vi "Begin.vi"(8 "error in":errorcluster) -> (0 "error out":errorcluster)   [LabVIEW 2018]
doc: "Called before other user functions, this VI can be used to open I/O refnums, load in file data, and do general program initialization. Notice that the <B>error out</B> terminal is simply used for data flow. Wiring it to other structures or subVIs ensures that this VI runs first."
uses:
  <vilib>/Rock Robotics/WPI/DriverStation/WPI_DriverStationRobotMode2.ctl
  <vilib>/Rock Robotics/WPI/Joystick/WPI_JoystickDeviceEnum.ctl
  <vilib>/Rock Robotics/WPI/SafetyOutput/WPI_SafetyOutputConfigMenu.ctl
  <vilib>/Rock Robotics/WPI/Solenoid/WPI_SolenoidChannel.ctl
  Robot Global Data.vi
  <vilib>/Rock Robotics/Network Tables/NT Write String Array.vi
  <vilib>/Rock Robotics/WPI/RobotDrive/WPI_RobotDriveOpen4MotorWithExistingMotors.vi
  <vilib>/Rock Robotics/WPI/Solenoid/WPI_SolenoidOpenSingle.vi
  <vilib>/Rock Robotics/WPI/Solenoid/WPI_SolenoidOpenDouble.vi
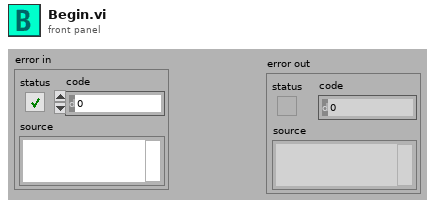
[diagram p1: front panel]
types:
  T1 = typedef "WPI_SafetyOutputConfigMenu.ctl" = enum16{"Enable", "Disable"}
  T2 = typedef "WPI_JoystickDeviceEnum.ctl" = enum16{"USB 0", "USB 1", "USB 2", "USB 3", "USB 4", "USB 5"}
  T3 = typedef "WPI_DriverStationRobotMode2.ctl" = enum16{"Autonomous Disabled", "Autonomous Enabled", "Teleop Disabled", "Teleop Enabled", "Disconnected", "Finish", "Test Disabled", "Test Enabled", "Emergency Stopped"}
  T4 = typedef "WPI_SolenoidChannel.ctl" = enum8{"Solenoid 0", "Solenoid 1", "Solenoid 2", "Solenoid 3", "Solenoid 4", "Solenoid 5", "Solenoid 6", "Solenoid 7", "Invalid"}
  T5 = typedef "WPI_SolenoidDevRef.ctl" = cluster{"DevStatus":errorcluster, "Pneumatics Control Module":u8, "Forward Solenoid Channel":T4, "Reverse Solenoid Channel":T4}
  T6 = typedef "WPI_CompressorDevRef.ctl" = cluster{"DevStatus":errorcluster, "Pneumatics Control Module":u8}
  T7 = typedef "WPI_MotorControlDeviceRef.ctl" = cluster{"DeviceStatus":errorcluster, "Type":T8, "PWM":cluster{"PWM Channel":T9, "DeadBand":T10}, "CAN":cluster{"Device Number":u8, "SetOutput VI Ref":variant, "GetOutput VI Ref":variant, "Enable VI Ref":variant, "Disable VI Ref":variant, "Data":variant}, "Invert":bool, "DIO PWM":cluster{"PWM \"Enable\" Channel":T9, "DIOChannel":T11, "PWM Rate":dbl}}
  T8 = typedef "WPI_MotorControlType.ctl" = enum16{"PWM", "CAN", "DIO PWM"}
  T9 = typedef "FPGA_DIOPWMChannel.ctl" = enum8{"PWM 0", "PWM 1", "PWM 2", "PWM 3", "PWM 4", "PWM 5", "PWM 6", "PWM 7", "PWM 8", "PWM 9", "PWM MXP 0", "PWM MXP 1", "PWM MXP 2", "PWM MXP 3", "PWM MXP 4", "PWM MXP 5", "PWM MXP 6", "PWM MXP 7", "PWM MXP 8", "PWM MXP 9", "Invalid"}
  T10 = typedef "WPI_PWMDeadband.ctl" = cluster{"Name":string, "maxPositivePwm":i32, "minPositivePwm":i32, "centerPwm":i32, "maxNegativePwm":i32, "minNegativePwm":i32, "angularRange":u16}
  T11 = typedef "FPGA_DIOChannel.ctl" = enum8{"DIO 0", "DIO 1", "DIO 2", "DIO 3", "DIO 4", "DIO 5", "DIO 6", "DIO 7", "DIO 8", "DIO 9", "DIO MXP 0", "DIO MXP 1", "DIO MXP 2", "DIO MXP 3", "DIO MXP 4", "DIO MXP 5", "DIO MXP 6", "DIO MXP 7", "DIO MXP 8", "DIO MXP 9", "DIO MXP 10", "DIO MXP 11", "DIO MXP 12", "DIO MXP 13", "DIO MXP 14", "DIO MXP 15", "SPI Port CS1", "SPI Port CS2", "SPI Port CS3", "SPI Port MISO", "SPI Port MOSI", "Invalid"}
  T12 = typedef "WPI_JoystickDevRef.ctl" = cluster{"Device":T2}
  T13 = typedef "WPI_RobotDriveDevRef.ctl" = cluster{"DevStatus":errorcluster, "Motors[]":T7[], "Square Inputs":bool, "Max Output":dbl}
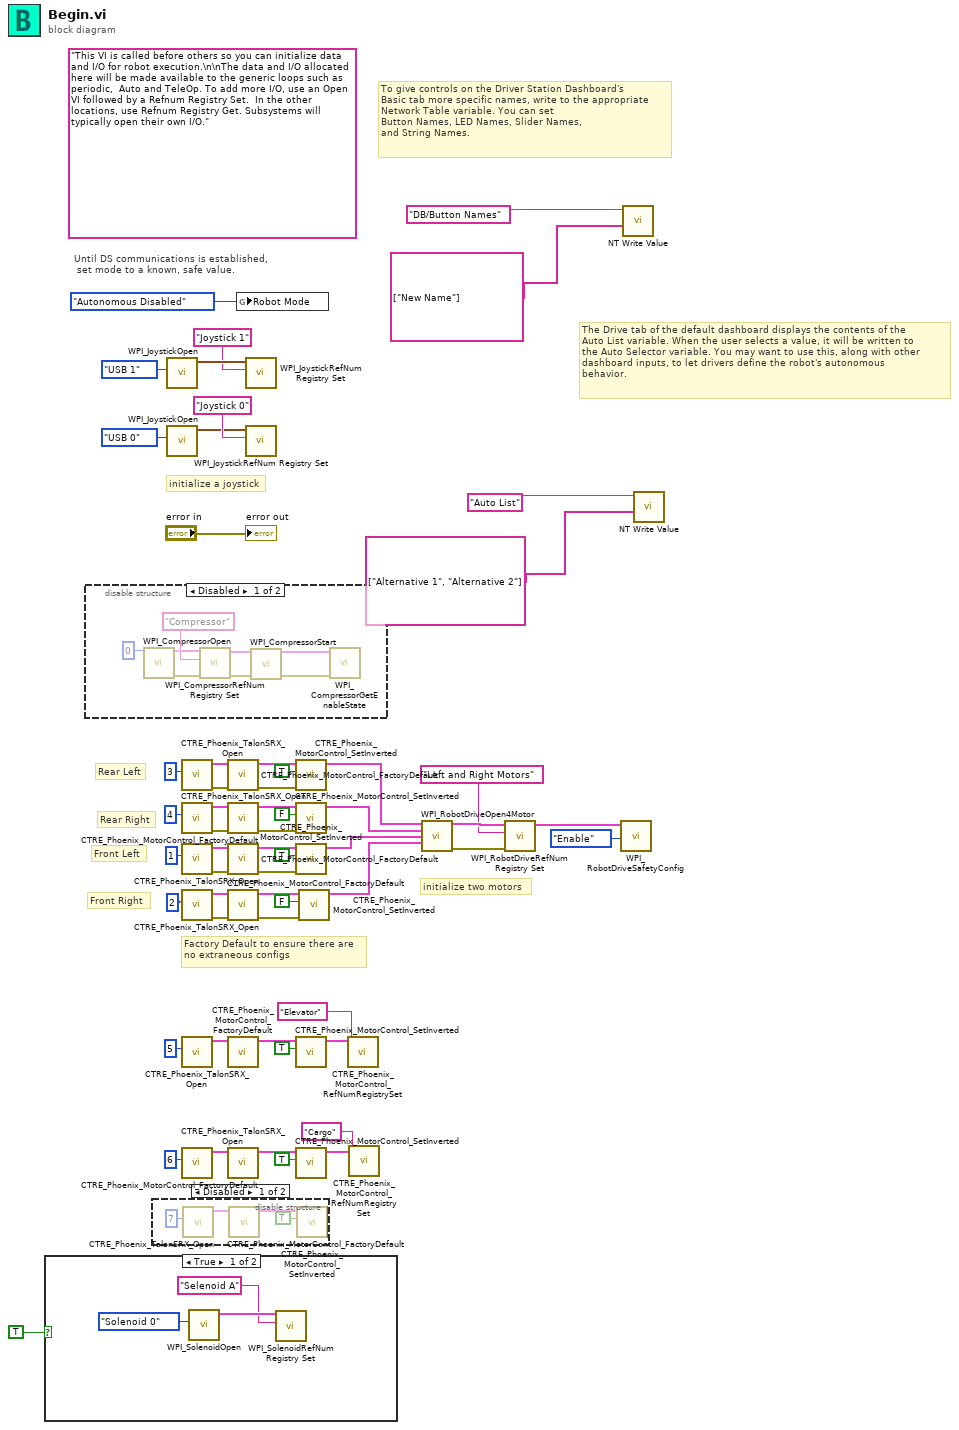
[diagram p0: block diagram]
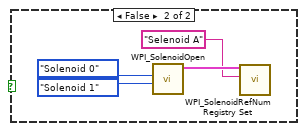
[diagram p2: hidden frame]
diagram:
  (unwired) "This VI is called before others so you can initialize data and I/O for robot execution.\n\nThe data and I/O allocated here will be made available to the generic loops such as periodic,  Auto and TeleOp. To add more I/O, use an Open VI followed by a Refnum Registry Set.  In the other locations, use Refnum Registry Get. Subsystems will typically open their own I/O."
  # "Factory Default to ensure there are\nno extraneous configs"
  # "Front Right"
  # "Front Left"
  # "Rear Right"
  # "Rear Left"
  # "initialize two motors"
  # "The Drive tab of the default dashboard displays the contents of the\nAuto List variable. When the user selects a value, it will be written to\nthe Auto Selector variable. You may want to use this, along with other\ndashboard inputs, to let drivers define the robot's autonomous\nbehavior."
  # "To give controls on the Driver Station Dashboard's\nBasic tab more specific names, write to the appropriate\nNetwork Table variable. You can set\nButton Names, LED Names, Slider Names,\nand String Names."
  # "initialize a joystick"
  # "Until DS communications is established,\n set mode to a known, safe value."
  n1 = case shown="True" TRUE {
    frame True {
      n2 = call-poly <vilib>:"WPI_SolenoidOpen.vi"("Solenoid Channel"=WPI_SolenoidChannel."Solenoid 0") -> ("SolenoidDevRef"=w60:T5)  [unwired: 9 in, 1 out]
      n3 = call <vilib>:"WPI_SolenoidRefNum Registry Set.vi"("refnum name"="Selenoid A", "SolenoidDevRef"=w60) -> ()  [unwired: 8 in, 2 out]
    }
    frame False {
      n4 = call-poly <vilib>:"WPI_SolenoidOpen.vi"("Reverse Solenoid Channel"=WPI_SolenoidChannel."Solenoid 1", "Forward Solenoid Channel"=WPI_SolenoidChannel."Solenoid 0" ("Solenoid Channel")) -> ("SolenoidDevRef"=w64:T5)  [unwired: 8 in, 1 out]
      n5 = call <vilib>:"WPI_SolenoidRefNum Registry Set.vi"("refnum name"="Selenoid A", "SolenoidDevRef"=w64) -> ()  [unwired: 8 in, 2 out]
    }
  }
  n6 = disable-structure shown="Disabled" {
    frame Disabled {
      n7 = call <vilib>:"WPI_CompressorOpen.vi"("Pneumatics Control Module (0)"=u8 0) -> ("CompressorDevRef"=w71:T6, "error out"=w68:errorcluster)  [unwired: 13 in]
      n8 = call <vilib>:"WPI_CompressorRefNum Registry Set.vi"("error in (no error)"=w68, "refnum name"="Compressor", "CompressorDevRef"=w71) -> ("error out"=w69:errorcluster, "CompressorDevRef"=w70:T6)  [unwired: 7 in]
      n9 = call <vilib>:"WPI_CompressorStart.vi"("error in (no error)"=w69, "CompressorDevRef"=w70) -> ("error out"=w66:errorcluster, "CompressorDevRef"=w67:T6)  [unwired: 8 in]
      n10 = call <vilib>:"WPI_CompressorGetEnableState.vi"("error in (no error)"=w66, "CompressorDevRef"=w67) -> ()  [unwired: 6 in, 4 out]
    }
    frame Enabled {
    }
  }
  n11 = disable-structure shown="Disabled" {
    frame Disabled {
      n12 = call <vilib>:"CTRE_Phoenix_TalonSRX_Open.vi"("Device Number"=u8 7) -> ("CAN Talon SRX Ref"=w76:T7)  [unwired: 9 in, 1 out]
      n13 = call <vilib>:"CTRE_Phoenix_MotorControl_FactoryDefault.vi"("PhoenixMotorControlDevRef"=w76) -> ("PhoenixMotorControlDevRef"=w77:T7)  [unwired: 9 in, 1 out]
      n14 = call <vilib>:"CTRE_Phoenix_MotorControl_SetInverted.vi"("Invert?"=TRUE, "PhoenixMotorControlDevRef"=w77) -> ()  [unwired: 8 in, 2 out]
    }
    frame Enabled {
    }
  }
  n15 = call <vilib>:"WPI_JoystickOpen.vi"("JoystickDevice"=WPI_JoystickDeviceEnum."USB 1") -> ("JoystickDevRef"=w48:T12)  [unwired: 10 in]
  n16 = call <vilib>:"WPI_JoystickOpen.vi"("JoystickDevice"=WPI_JoystickDeviceEnum."USB 0") -> ("JoystickDevRef"=w56:T12)  [unwired: 10 in]
  n17 = call <vilib>:"CTRE_Phoenix_TalonSRX_Open.vi"("Device Number"=u8 3) -> ("error out"=w29:errorcluster, "CAN Talon SRX Ref"=w28:T7)  [unwired: 9 in]
  n18 = call <vilib>:"CTRE_Phoenix_TalonSRX_Open.vi"("Device Number"=u8 4) -> ("error out"=w27:errorcluster, "CAN Talon SRX Ref"=w26:T7)  [unwired: 9 in]
  n19 = call <vilib>:"CTRE_Phoenix_TalonSRX_Open.vi"("Device Number"=u8 1) -> ("error out"=w25:errorcluster, "CAN Talon SRX Ref"=w24:T7)  [unwired: 9 in]
  n20 = call <vilib>:"CTRE_Phoenix_TalonSRX_Open.vi"("Device Number"=u8 2) -> ("error out"=w23:errorcluster, "CAN Talon SRX Ref"=w22:T7)  [unwired: 9 in]
  n21 = call <vilib>:"CTRE_Phoenix_TalonSRX_Open.vi"("Device Number"=u8 5) -> ("CAN Talon SRX Ref"=w5:T7)  [unwired: 9 in, 1 out]
  n22 = call <vilib>:"CTRE_Phoenix_TalonSRX_Open.vi"("Device Number"=u8 6) -> ("CAN Talon SRX Ref"=w11:T7)  [unwired: 9 in, 1 out]
  n23 = call <vilib>:"CTRE_Phoenix_MotorControl_FactoryDefault.vi"("error in"=w29, "PhoenixMotorControlDevRef"=w28) -> ("error out"=w20:errorcluster, "PhoenixMotorControlDevRef"=w21:T7)  [unwired: 8 in]
  n24 = call <vilib>:"CTRE_Phoenix_MotorControl_FactoryDefault.vi"("error in"=w27, "PhoenixMotorControlDevRef"=w26) -> ("error out"=w18:errorcluster, "PhoenixMotorControlDevRef"=w19:T7)  [unwired: 8 in]
  n25 = call <vilib>:"CTRE_Phoenix_MotorControl_FactoryDefault.vi"("error in"=w25, "PhoenixMotorControlDevRef"=w24) -> ("error out"=w16:errorcluster, "PhoenixMotorControlDevRef"=w17:T7)  [unwired: 8 in]
  n26 = call <vilib>:"CTRE_Phoenix_MotorControl_FactoryDefault.vi"("error in"=w23, "PhoenixMotorControlDevRef"=w22) -> ("error out"=w14:errorcluster, "PhoenixMotorControlDevRef"=w15:T7)  [unwired: 8 in]
  n27 = call <vilib>:"CTRE_Phoenix_MotorControl_FactoryDefault.vi"("PhoenixMotorControlDevRef"=w5) -> ("PhoenixMotorControlDevRef"=w6:T7)  [unwired: 9 in, 1 out]
  n28 = call <vilib>:"CTRE_Phoenix_MotorControl_FactoryDefault.vi"("PhoenixMotorControlDevRef"=w11) -> ("PhoenixMotorControlDevRef"=w10:T7)  [unwired: 9 in, 1 out]
  n29 = global write "Robot Global Data.vi" "Robot Mode"(WPI_DriverStationRobotMode2."Autonomous Disabled" ("Robot Mode")) -> ()
  n30 = call <vilib>:"WPI_JoystickRefNum Registry Set.vi"("refnum name"="Joystick 1", "JoystickDevRef"=w48) -> ()  [unwired: 8 in, 2 out]
  n31 = call <vilib>:"WPI_JoystickRefNum Registry Set.vi"("refnum name"="Joystick 0", "JoystickDevRef"=w56) -> ()  [unwired: 8 in, 2 out]
  n32 = call <vilib>:"CTRE_Phoenix_MotorControl_SetInverted.vi"("error in (no error)"=w20, "Invert?"=TRUE, "PhoenixMotorControlDevRef"=w21) -> ("PhoenixMotorControlDevRef"=w30:T7)  [unwired: 7 in, 1 out]
  n33 = call <vilib>:"CTRE_Phoenix_MotorControl_SetInverted.vi"("error in (no error)"=w18, "Invert?"=FALSE, "PhoenixMotorControlDevRef"=w19) -> ("PhoenixMotorControlDevRef"=w35:T7)  [unwired: 7 in, 1 out]
  n34 = call <vilib>:"CTRE_Phoenix_MotorControl_SetInverted.vi"("error in (no error)"=w16, "Invert?"=TRUE, "PhoenixMotorControlDevRef"=w17) -> ("PhoenixMotorControlDevRef"=w32:T7)  [unwired: 7 in, 1 out]
  n35 = call <vilib>:"CTRE_Phoenix_MotorControl_SetInverted.vi"("Invert?"=TRUE, "PhoenixMotorControlDevRef"=w6) -> ("PhoenixMotorControlDevRef"=w2:T7)  [unwired: 8 in, 1 out]
  n36 = call <vilib>:"CTRE_Phoenix_MotorControl_SetInverted.vi"("Invert?"=TRUE, "PhoenixMotorControlDevRef"=w10) -> ("PhoenixMotorControlDevRef"=w9:T7)  [unwired: 8 in, 1 out]
  n37 = call <vilib>:"CTRE_Phoenix_MotorControl_SetInverted.vi"("error in (no error)"=w14, "Invert?"=FALSE, "PhoenixMotorControlDevRef"=w15) -> ("PhoenixMotorControlDevRef"=w37:T7)  [unwired: 7 in, 1 out]
  n38 = call <vilib>:"CTRE_Phoenix_MotorControl_RefNumRegistrySet.vi"("refnum name"="Elevator", "PhoenixMotorControlDevRef"=w2) -> ()  [unwired: 8 in, 2 out]
  n39 = call <vilib>:"CTRE_Phoenix_MotorControl_RefNumRegistrySet.vi"("refnum name"="Cargo", "PhoenixMotorControlDevRef"=w9) -> ()  [unwired: 8 in, 2 out]
  n40 = call-poly <vilib>:"WPI_RobotDriveOpen4Motor.vi"("Rear Left Motor Dev Ref"=w30, "Rear Right Motor Dev Ref"=w35, "Front Left Motor Dev Ref"=w32, "Front Right Motor Dev Ref"=w37) -> ("RobotDriveDevRef"=w46:T13, "error out"=w44:errorcluster)  [unwired: 10 in]
  n41 = call <vilib>:"WPI_RobotDriveRefNum Registry Set.vi"("error in (no error)"=w44, "refnum name"="Left and Right Motors", "RobotDriveDevRef"=w46) -> ("RobotDriveDevRef"=w43:T13)  [unwired: 1 in, 7 out]
  n42 = call <vilib>:"WPI_RobotDriveSafetyConfig.vi"("mode"=WPI_SafetyOutputConfigMenu."Enable", "RobotDriveDevRef"=w43) -> ()  [unwired: 8 in, 2 out]
  n43 = call-poly <vilib>:"NT Write Value.vi"("String Array"=string[] ["New Name"], "Name"="DB/Button Names") -> ()  [unwired: 9 in, 1 out]
  n44 = call-poly <vilib>:"NT Write Value.vi"("String Array"=string[] ["Alternative 1", "Alternative 2"], "Name"="Auto List") -> ()  [unwired: 9 in, 1 out]
  "error out" <- "error in"
